vi "Add Lines From Database.vi"(8 "error in":errorcluster, 11 "Objects":T1) -> (0 "error out":errorcluster, 1 "Success?":bool, 2 "Line Index":i32)   [LabVIEW 2017, in "J1939 editor node.lvclass"]
uses:
  J1939 editor node.lvclass
  <vilib>/NI/DCAF/Tag Editor Core/Table API/Table Manager/object ref.ctl
  <vilib>/NI/DCAF/Tag Editor Core/Configuration Editor/Classes/Engine Parent/Engine Parent Editor Node.lvclass
  <vilib>/NI/DCAF/Tag Editor Core/Configuration Editor/Classes/Module editor node/module editor node.lvclass
  <vilib>/NI/Tag Bus Module Framework/channel/channel classification.ctl
  <vilib>/NI/Tag Bus Module Framework/channel/TBM channel.lvclass
  <resource>/objmgr/xnet.rc
  <vilib>/NI/DCAF/Tag Editor Core/Table API/Table Manager/Table Manager.lvclass
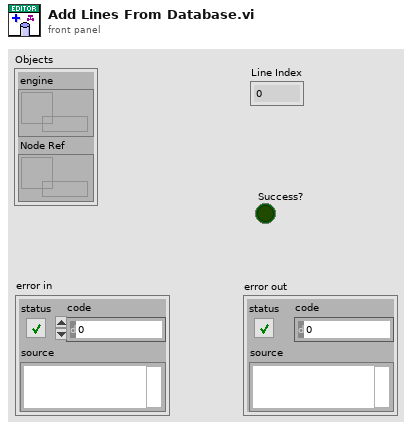
[diagram p1: front panel]
types:
  T1 = typedef "Table Manager.lvlib/Table Manager.lvclass/object ref.ctl" = cluster{"engine":refnum<data-value>, "Node Ref":refnum<data-value>}
  T2 = typedef "TBM channel.lvclass/channel classification.ctl" = enum16{"input data", "output data", "processing parameter", "processing result"}
  T3 = typedef "J1939 editor node.lvclass/Mappings.ctl" = cluster{"Line":T4, "Maps":T5[]}
  T4 = typedef "J1939 configuration.lvclass/Line.ctl" = cluster{"channel":refnum<class "TBM channel.lvclass">, "XNET Signal":refnum<k21>}
  T5 = typedef "J1939 editor node.lvclass/Map.ctl" = cluster{"channel":refnum<class "TBM channel.lvclass">, "tag name":string}
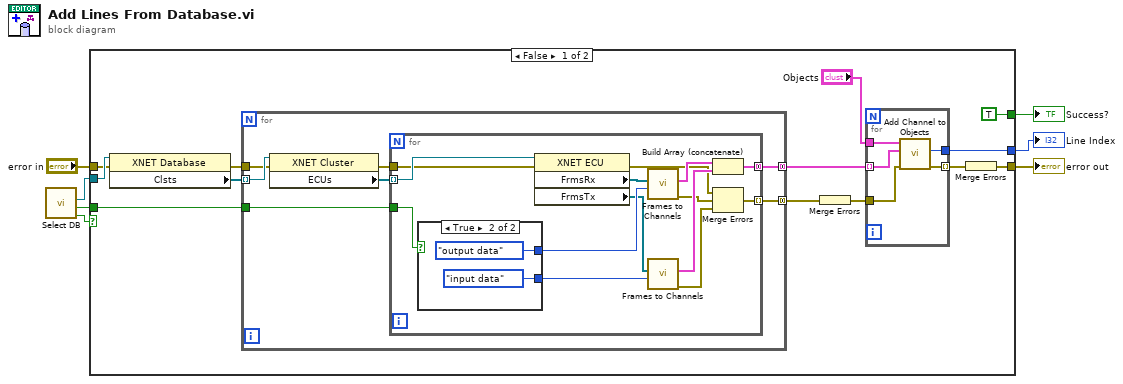
[diagram p0: block diagram]
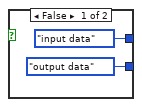
[diagram p2: hidden frame]
diagram:
  n1 = call "Select DB.vi"() -> ("Cancel out"=w5:bool, "Invert Channels out"=w6:bool, "XNET Database out"=w7:refnum<k21>)  [unwired: 9 in]
  n2 = case shown="False" w5 {
    tunnel: w7 -> [w20 _]
    tunnel: w6 -> [w18 _]
    tunnel: "error in" -> [w17 w51]
    tunnel: [TRUE _] -> w1
    tunnel: [w9 w51] -> w2
    tunnel: [w11 _] -> w3
    frame False {
      n3 = property class="XNET Database"(reference=w20, error in=w17) -> (error out=w16:errorcluster, "Clsts"=w19:refnum<k21>[])  [unwired: 1 out]
      n4 = for {
        tunnel: w19 -> [w32] mode=indexing
        tunnel: w18 -> [w30]
        tunnel: [w29] -> w13 mode=concatenating
        tunnel: w16 -> [w28]
        tunnel: [w26] -> w12 mode=concatenating
        n5 = property class="XNET Cluster"(reference=w32, error in=w28) -> (error out=w27:errorcluster, "ECUs"=w31:refnum<k21>[])  [unwired: 1 out]
        n6 = for {
          tunnel: w31 -> [w45] mode=indexing
          tunnel: w30 -> [w46]
          tunnel: [w38] -> w29 mode=concatenating
          tunnel: w27 -> [w37]
          tunnel: [w36] -> w26 mode=indexing
          n7 = case shown="True" w46 {
            tunnel: [channel_classification."input data" ("channel classification") channel_classification."output data" ("channel classification")] -> w43
            tunnel: [channel_classification."output data" ("channel classification") channel_classification."input data" ("channel classification")] -> w41
            frame False {
            }
            frame True {
            }
          }
          n8 = property class="XNET ECU"(reference=w45, error in=w37) -> (error out=w35:errorcluster, "FrmsRx"=w44:refnum<k21>[], "FrmsTx"=w42:refnum<k21>[])  [unwired: 1 out]
          n9 = call "Frames to Channels.vi"("channel classification"=w43, "Frames"=w44) -> ("error out"=w33:errorcluster, "Mappings out"=w40:T3[])  [unwired: 8 in]
          n10 = call "Frames to Channels.vi"("channel classification"=w41, "Frames"=w42) -> ("error out"=w34:errorcluster, "Mappings out"=w39:T3[])  [unwired: 8 in]
          n11 = Build Array (concatenate)(w40, w39) -> (w38:T3[])
          n12 = Merge Errors(w35, w33, w34) -> (w36:errorcluster)
        }
      }
      n13 = Merge Errors(w12) -> (w14:errorcluster)
      n14 = for {
        tunnel: "Objects" -> [w23]
        tunnel: w13 -> [w22] mode=indexing
        tunnel: w14 -> [w24]
        tunnel: [w25] -> w10 mode=indexing
        tunnel: [w21] -> w11
        n15 = call "Add Channel to Objects.vi"("error in"=w24, "Line Item in"=w22, "Objects in"=w23) -> ("error out"=w25:errorcluster, "Line Index"=w21:i32)  [unwired: 7 in]
      }
      n16 = Merge Errors(w10) -> (w9:errorcluster)
    }
    frame True {
    }
  }
  "Success?" <- w1
  "error out" <- w2
  "Line Index" <- w3
